vi "historic_stock.vi"() -> ()   [LabVIEW 8.6]
uses:
  <vilib>/httpClient/LabVIEWHTTPClient.lvlib
panel:
  out "Status":string
  in  "Exchange":string(combo)
  in  "SYMBOL":string
  out "XY Graph":cluster{timestamp, dbl}[](graph)
  in  "stop":bool
  in  "Refresh Quote":bool
  # "Historic Stock Prices"
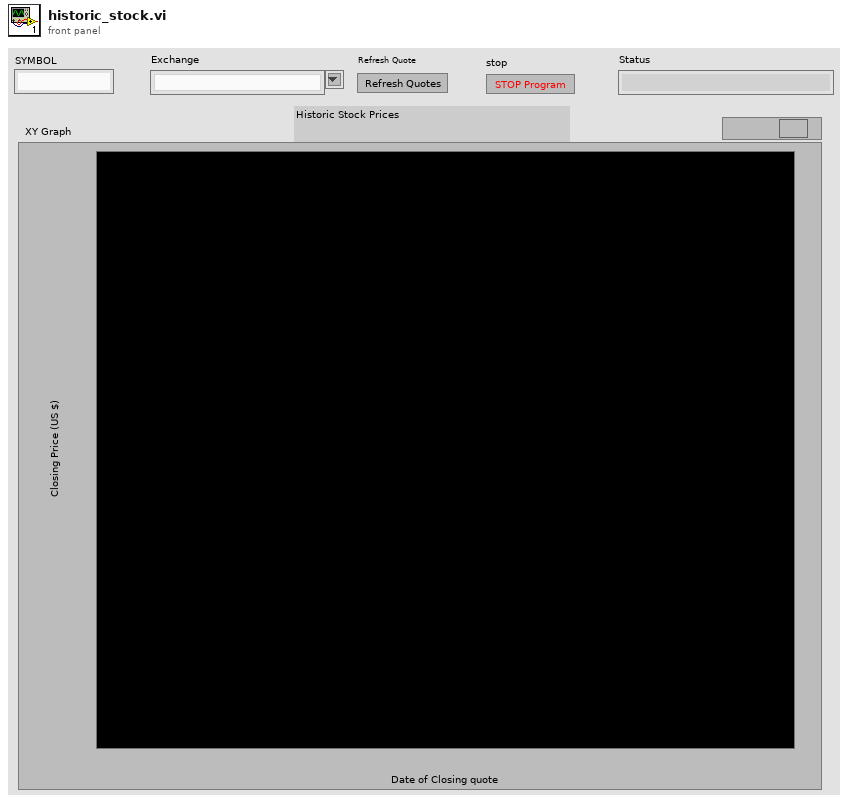
[diagram p1: front panel]
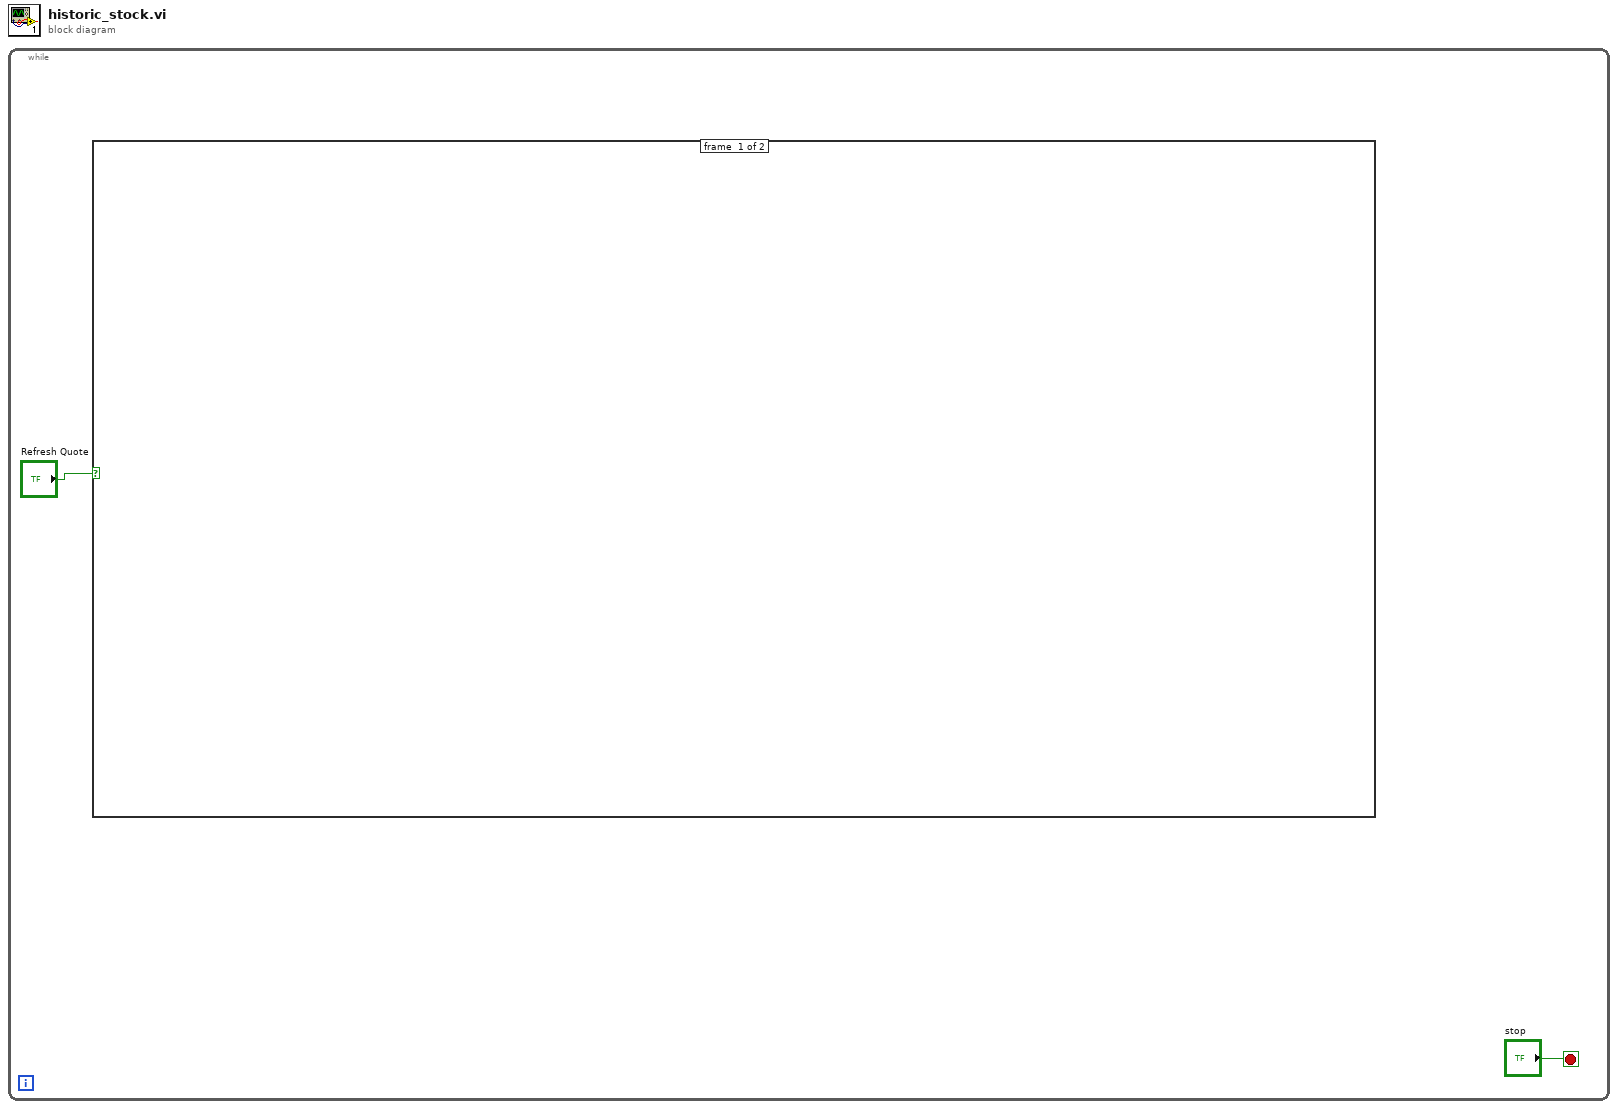
[diagram p0: block diagram]
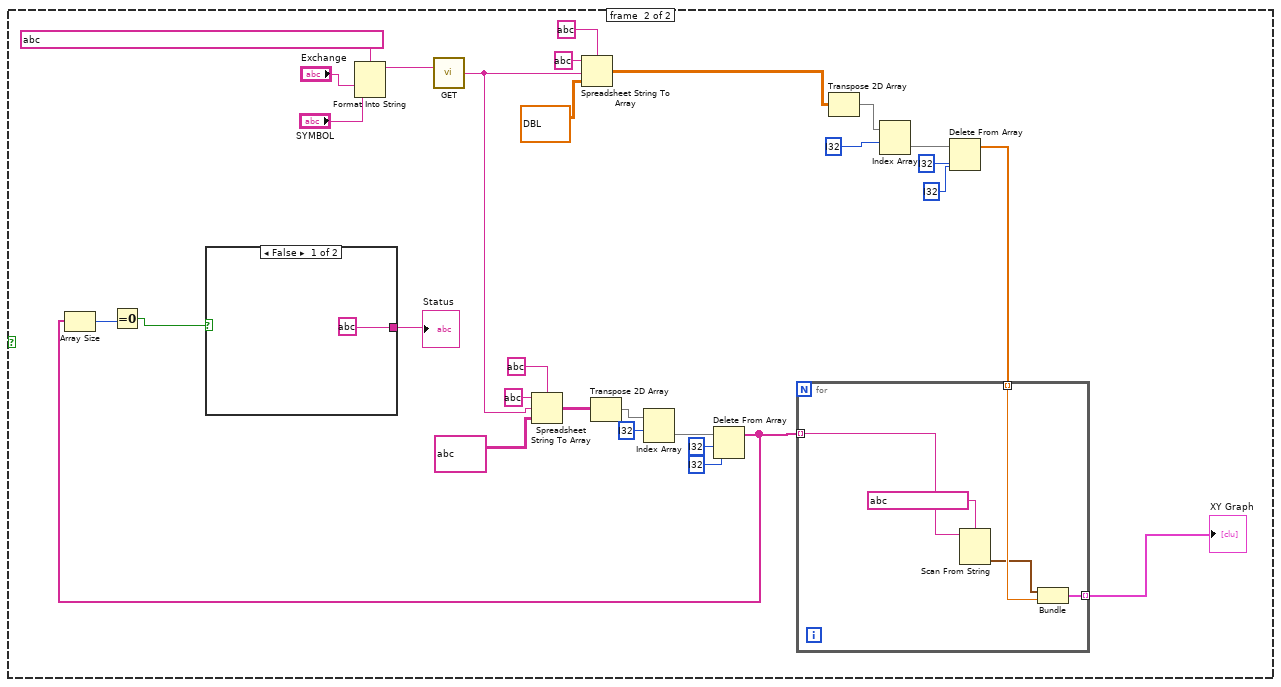
[diagram p2: hidden frame]
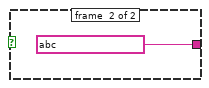
[diagram p3: hidden frame]
diagram:
  n1 = while {
    stop <- "stop" stop-if-true
    n2 = case shown="True" "Refresh Quote" {
      frame #0 {
      }
      frame #1 {
        n3 = Format Into String(format string=string ?, "Exchange", "SYMBOL") -> (resulting string=w22:string)  [unwired: 2 in, 1 out]
        n4 = call <vilib>:"GET.vi"("url"=w22) -> ("body"=w8:string)  [unwired: 11 in, 3 out]
        n5 = Spreadsheet String To Array(delimiter (Tab)=string ?, format string=string ?, spreadsheet string=w8, array type (2D Dbl)=string[][] ? ("Array")) -> (array=w18:string[][])
        n6 = Spreadsheet String To Array(delimiter (Tab)=string ?, format string=string ?, spreadsheet string=w8, array type (2D Dbl)=dbl[][] ?) -> (array=w7:dbl[][])
        n7 = Transpose 2D Array(2D array=w18) -> (transposed array=w17:string[][])
        n8 = Index Array(array=w17, index (row)=i32 ?) -> (element=w15:string[])  [unwired: 1 in]
        n9 = Delete From Array(array=w15, length=i32 ?, index=i32 ?) -> (array with subset deleted=w4:string[])  [unwired: 1 out]
        n10 = Array Size(array=w4) -> (size(s)=w6:i32)
        n11 = Equal To 0?(x=w6) -> (x = 0?=w5:bool)
        n12 = case shown="False" w5 {
          tunnel: [string ? ("Status") string ? ("Status")] -> w3
          frame #0 {
          }
          frame #1 {
          }
        }
        "Status" <- w3
        n13 = Transpose 2D Array(2D array=w7) -> (transposed array=w27:dbl[][])
        n14 = Index Array(array=w27, index (row)=i32 ?) -> (element=w26:dbl[])  [unwired: 1 in]
        n15 = Delete From Array(array=w26, length=i32 ?, index=i32 ?) -> (array with subset deleted=w12:dbl[])  [unwired: 1 out]
        n16 = for {
          tunnel: w4 -> [w38] mode=indexing
          tunnel: w12 -> [w36] mode=indexing
          tunnel: [w35] -> w11 mode=indexing
          n17 = Scan From String(format string=string ?, input string=w38) -> (output 1=w34:timestamp)  [unwired: 3 in, 3 out]
          n18 = Bundle(w34, w36) -> (w35:cluster{timestamp, dbl})  [unwired: 1 in]
        }
        "XY Graph" <- w11
      }
    }
  }
